vi "Interface2.vi"() -> ()   [LabVIEW 2010]
panel:
  in  "退出":bool
  in  "读数据":bool
  out "数据":dbl
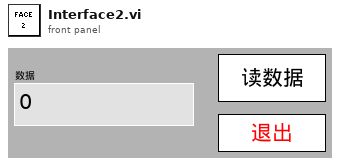
[diagram p1: front panel]
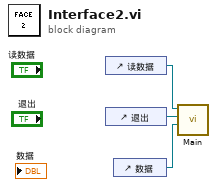
[diagram p0: block diagram]
diagram:
  n1 = control-ref of="读数据"() -> (w3:refnum<vi>)
  n2 = control-ref of="退出"() -> (w2:refnum<vi>)
  n3 = control-ref of="数据"() -> (w1:refnum<vi>)
  n4 = call "Main.vi"("numeric"=w1, "stop"=w2, "get value"=w3) -> ()  [unwired: 9 in]
